vi "Write TemperatureFieldRegression.vi"(8 "error in (no error)":errorcluster, 10 "TemperatureFieldRegression":dbl[][](array[numeric]), 11 "Temp params in":refnum<class "CV-Temperature.lvclass">) -> (0 "error out":errorcluster, 3 "Temp params out":refnum<class "CV-Temperature.lvclass">)   [LabVIEW 2013, in "CameraVision.lvlib" / "CV-Temperature.lvclass"]
uses:
  CV-Temperature.lvclass
  CV-Temperature.lvclass/CV-Temperature.ctl
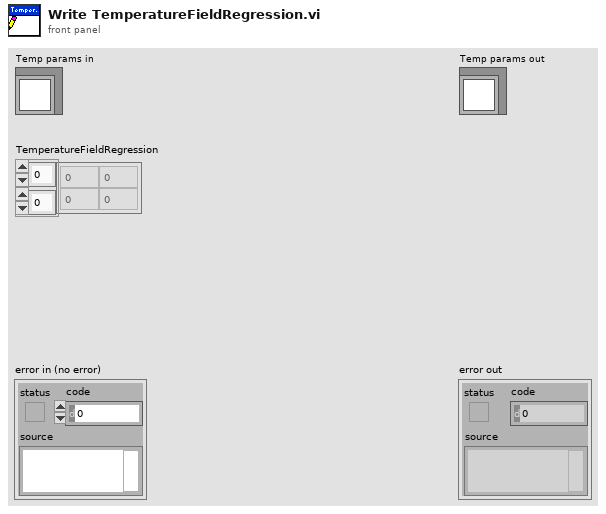
[diagram p1: front panel]
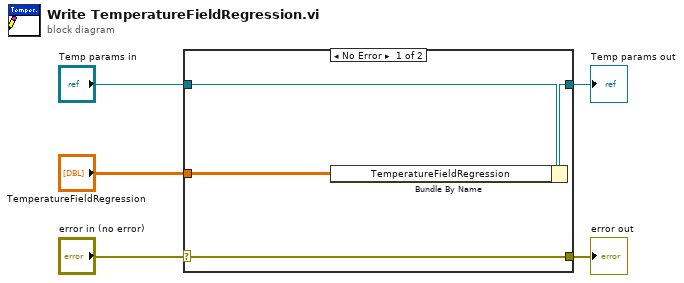
[diagram p0: block diagram]
diagram:
  n1 = case shown="No Error" "error in (no error)" {
    selector: "error in (no error)" -> [w9 w10]
    tunnel: [w9 w10] -> w4
    tunnel: [w7 w11] -> w2
    tunnel: "Temp params in" -> [w8 w11]
    tunnel: "TemperatureFieldRegression" -> [w6 _]
    frame No Error {
      n2 = Bundle By Name(cluster=w8, "TemperatureFieldRegression"=w6) -> (w7:refnum<class "CV-Temperature.lvclass">)
    }
    frame Error {
    }
  }
  "error out" <- w4
  "Temp params out" <- w2
